vi "Parse Tags - Inline Version.vi"(6 "New Tag Info (F)":bool, 8 "error in (no error)":errorcluster, 9 "[Tags]":string[](array[string]), 11 "Cluster of Controls":variant) -> (0 "error out":errorcluster, 1 "[Whole Tags]":string[](array[string]), 2 "[VData out]":variant[](array[variant]), 3 "[Parsed Tags]":T1[](array[typedef]))   [LabVIEW 2018]
doc: "Converts a variant cluster input and/or an array of references and/or an array of strings to an array of tag information as well as variant data.\nNote1: Empty variant data will be output for Array of Strings.\nNote2: The names/strings will be parsed for any text before the first space in order to find the tags\n\nIf an array of references is input, the VI uses these references to get tag names using the references controls' labels. \n\nIf a cluster of controls is input, each item in the cluster will be used for its label and value.\n\nIf just an array of strings is input, the string values will be used as tags and there will be void values output."
uses:
  Shared Controls/Parsed Tag Cluster.ctl
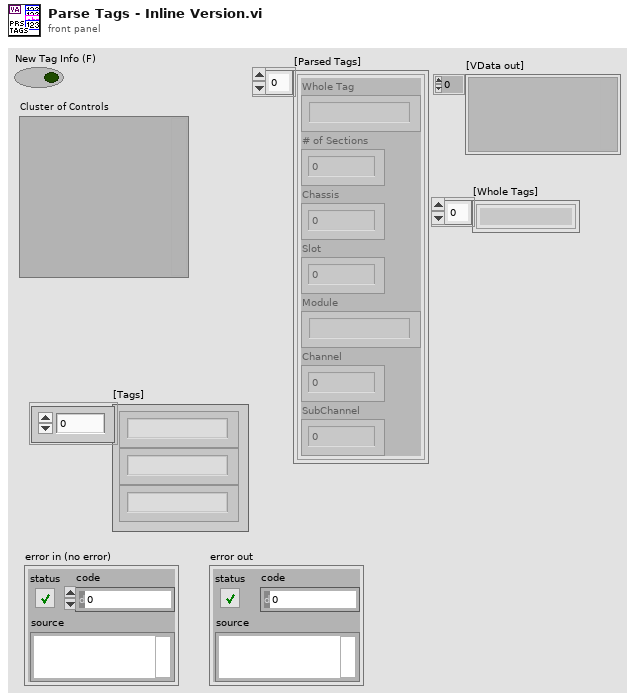
[diagram p1: front panel]
types:
  T1 = typedef "Parsed Tag Cluster.ctl" = cluster{"Whole Tag":string, "# of Sections":u8, "Chassis":u8, "Slot":u8, "Module":string, "Channel":u8, "SubChannel":u8}
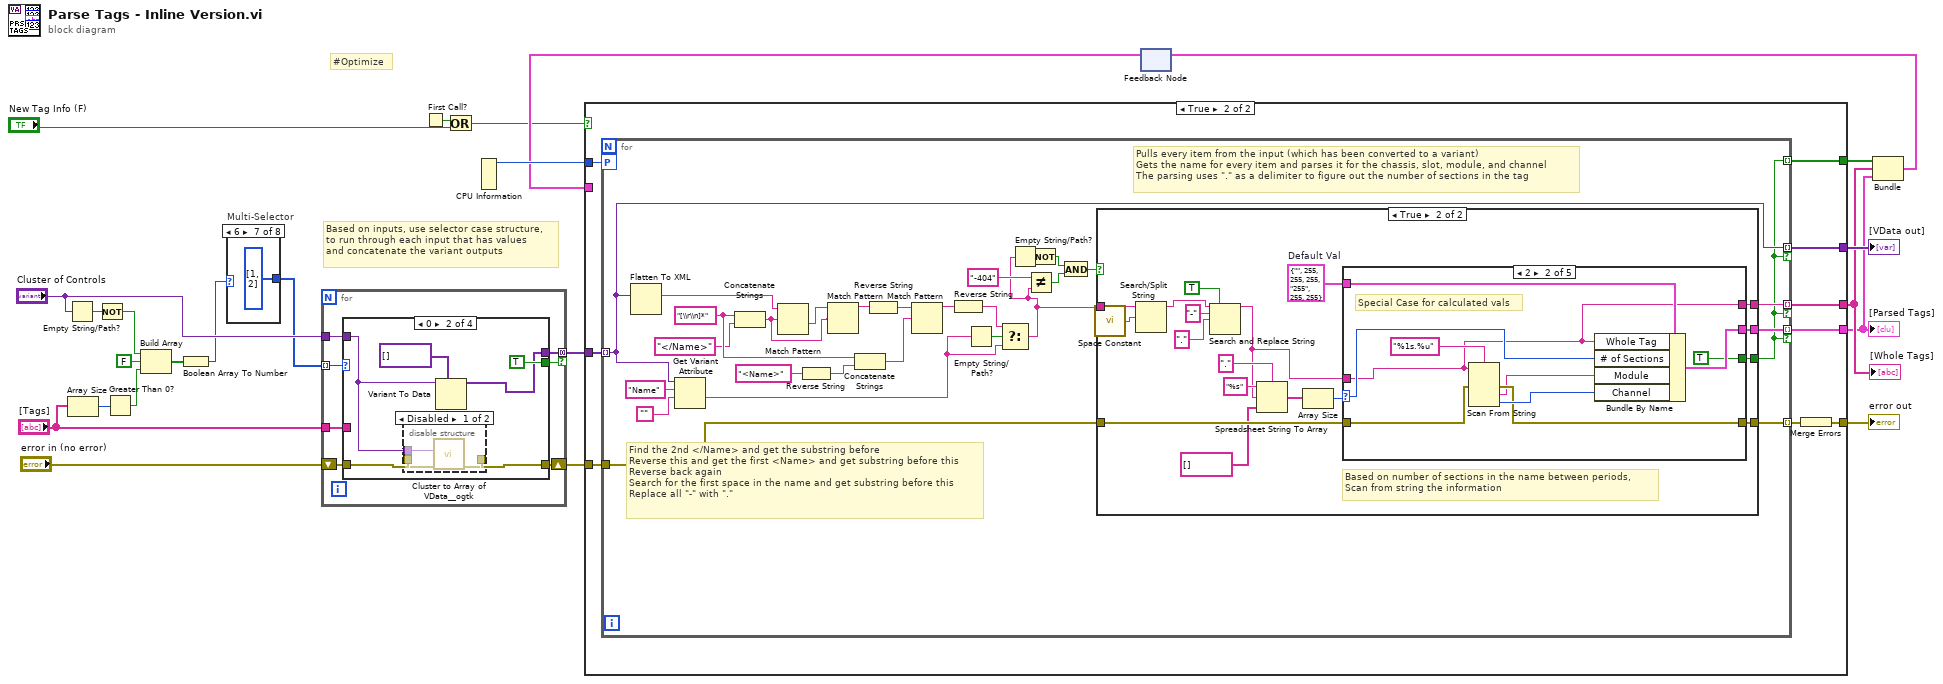
[diagram p0: block diagram]
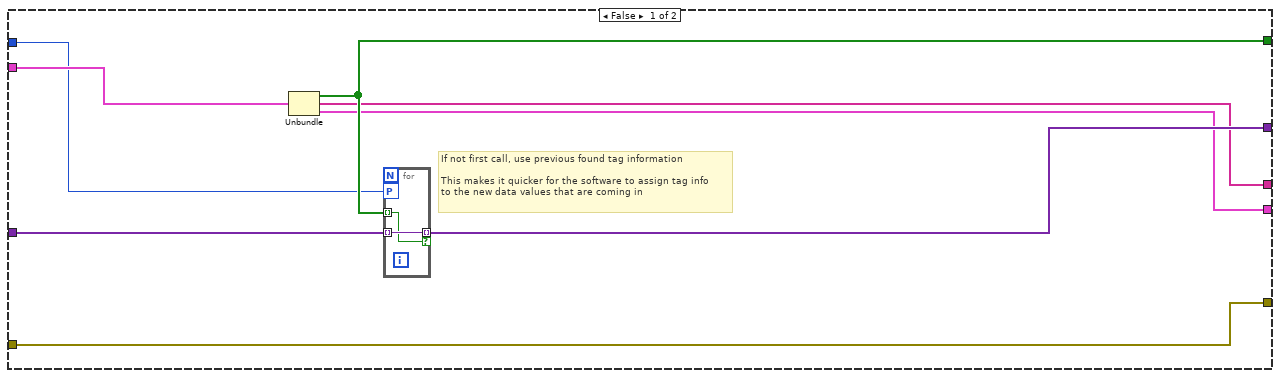
[diagram p2: hidden frame]
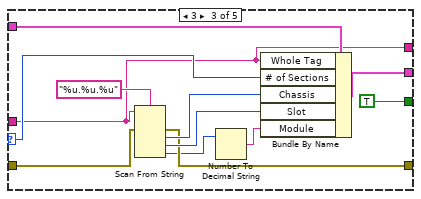
[diagram p5: hidden frame]
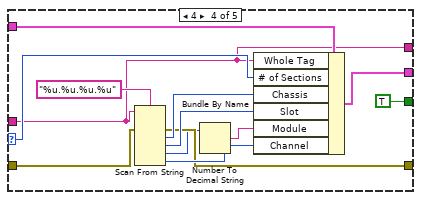
[diagram p6: hidden frame]
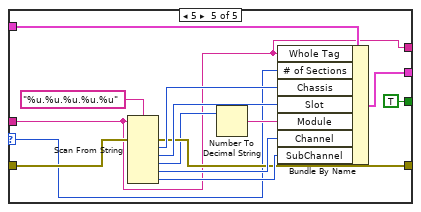
[diagram p7: hidden frame]
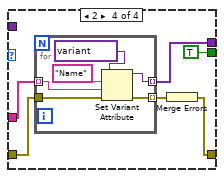
[diagram p11: hidden frame]
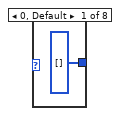
[diagram p12: hidden frame]
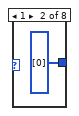
[diagram p13: hidden frame]
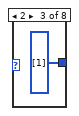
[diagram p14: hidden frame]
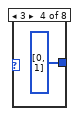
[diagram p15: hidden frame]
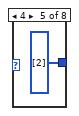
[diagram p16: hidden frame]
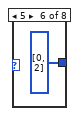
[diagram p17: hidden frame]
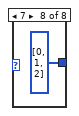
[diagram p18: hidden frame]
diagram:
  # "#Optimize"
  # "Based on inputs, use selector case structure,\nto run through each input that has values\nand concatenate the variant outputs"
  n1 = Empty String/Path?(string/path="Cluster of Controls") -> (empty?=w18:bool)
  n2 = Array Size(array="[Tags]") -> (size(s)=w22:i32)
  n3 = Not(x=w18) -> (.not. x?=w17:bool)
  n4 = Greater Than 0?(x=w22) -> (x > 0?=w21:bool)
  n5 = Build Array(w17, FALSE ("element"), w21) -> (w14:bool[])
  n6 = Boolean Array To Number(Boolean array=w14) -> (number=w16:u32)
  n7 = case "Multi-Selector" shown="6" w16 {
    tunnel: [u32[] [] u32[] [0] u32[] [1] u32[] [0, 1] u32[] [2] u32[] [0, 2] u32[] [1, 2] u32[] [0, 1, 2]] -> w15
    frame 0, Default {
    }
    frame 1 {
    }
    frame 2 {
    }
    frame 3 {
    }
    frame 4 {
    }
    frame 5 {
    }
    frame 6 {
    }
    frame 7 {
    }
  }
  n8 = for {
    tunnel: [w39] -> w24 mode=concatenating if=w33
    tunnel: "[Tags]" -> [w36]
    tunnel: "Cluster of Controls" -> [w35]
    tunnel: w15 -> [w34] mode=indexing
    shift-right: [w37] -> w1
    shift-left: "error in (no error)" -> [w38]
    n9 = case shown="0" w34 {
      tunnel: [_ w41 _ w56] -> w39
      tunnel: w38 -> [w40 w46 w50 w55]
      tunnel: [w40 w45 w50 w52] -> w37
      tunnel: w35 -> [_ w43 _ _]
      tunnel: w36 -> [_ _ _ w53]
      tunnel: [_ TRUE _ TRUE] -> w33
      frame Default {
      }
      frame 0 {
        n10 = disable-structure shown="Disabled" {
          disable-tunnel: w46 -> [w49 _]
          disable-tunnel: [w48 _] -> w45
          disable-tunnel: w43 -> [w47 _]
          frame Disabled {
            n11 = call <userlib>:"Cluster to Array of VData__ogtk.vi"("error in (no error)"=w49, "Cluster"=w47) -> ("error out"=w48:errorcluster)  [unwired: 8 in, 1 out]
          }
          frame Enabled {
          }
        }
        n12 = Variant To Data(type=variant[] [], Variant=w43) -> (data=w41:variant[])  [unwired: 1 in, 1 out]
      }
      frame 1 {
      }
      frame 2 {
        n13 = for {
          tunnel: [w59] -> w56 mode=indexing
          tunnel: w55 -> [w62]
          tunnel: [w61] -> w54 mode=indexing
          tunnel: w53 -> [w58] mode=indexing
          n14 = Set Variant Attribute(Variant=variant(string "TagOnly") ("variant"), name="Name", value=w58, error in=w62) -> (Variant out=w59:variant, error out=w61:errorcluster)  [unwired: 1 out]
        }
        n15 = Merge Errors(w54) -> (w52:errorcluster)
      }
    }
  }
  n16 = First Call?() -> (First Call?: T/F=w11:bool)
  n17 = Or(x=w11, y="New Tag Info (F)") -> (x .or. y?=w5:bool)
  n18 = CPU Information() -> (4:w13:i32)  [unwired: 3 out]
  n19 = feedback #1() -> (w9:cluster{bool[], string[], T1[]})  [unwired: 1 in]
  n20 = case shown="True" w5 {
    tunnel: [w65 w81] -> w6
    tunnel: [w63 w73] -> w3
    tunnel: w24 -> [w70 w80]
    tunnel: w1 -> [w63 w79]
    tunnel: [w69 w78] -> w23
    tunnel: [w66 w77] -> w7
    tunnel: w13 -> [w64 w76]
    tunnel: w9 -> [w68 _]
    tunnel: [w67 w75] -> w10
    frame False {
      # "If not first call, use previous found tag information\n\nThis makes it quicker for the software to assign tag info\nto the new data values that are coming in"
      n21 = Unbundle(w68) -> (w67:bool[], w66:string[], w65:T1[])
      n22 = for {
        tunnel: w70 -> [w72] mode=indexing
        tunnel: [w72] -> w69 mode=indexing if=w71
        tunnel: w67 -> [w71] mode=indexing
        workers-P: w64 -> [_]
      }
    }
    frame True {
      n23 = for {
        tunnel: [w107] -> w81 mode=indexing if=w82
        tunnel: w80 -> [w95] mode=indexing
        tunnel: w79 -> [w109]
        tunnel: [w108] -> w74 mode=indexing
        tunnel: [w95] -> w78 mode=indexing if=w82
        tunnel: [w89] -> w77 mode=indexing if=w82
        workers-P: w76 -> [_]
        tunnel: [w82] -> w75 mode=indexing
        w105 = "[\\r\\n]*"
        # "Find the 2nd </Name> and get the substring before\nReverse this and get the first <Name> and get substring before this\nReverse back again\nSearch for the first space in the name and get substring before this\nReplace all \"-\" with \".\""
        # "Pulls every item from the input (which has been converted to a variant)\nGets the name for every item and parses it for the chassis, slot, module, and channel\nThe parsing uses \".\" as a delimiter to figure out the number of sections in the tag"
        n24 = Flatten To XML(anything=w95) -> (xml string=w102:string)
        n25 = Get Variant Attribute(Variant=w95, name="Name", default value (empty Variant)="") -> (value=w90:string)  [unwired: 1 in, 3 out]
        n26 = Concatenate Strings(w105, "</Name>" ("Substring")) -> (w98:string)
        n27 = Match Pattern(string=w102, regular expression=w98) -> (after substring=w99:string)  [unwired: 1 in, 3 out]
        n28 = Reverse String(1:"<Name>") -> (0:w104:string)
        n29 = Match Pattern(string=w99, regular expression=w98) -> (before substring=w97:string)  [unwired: 1 in, 3 out]
        n30 = Concatenate Strings(w105, w104) -> (w106:string)
        n31 = Reverse String(1:w97) -> (0:w103:string)
        n32 = Match Pattern(string=w103, regular expression=w106) -> (before substring=w96:string)  [unwired: 1 in, 3 out]
        n33 = Reverse String(1:w96) -> (0:w91:string)
        n34 = Empty String/Path?(string/path=w90) -> (empty?=w92:bool)
        n35 = Select(t=w91, s=w92, f=w90) -> (s? t:f=w84:string)
        n36 = Empty String/Path?(string/path=w84) -> (empty?=w86:bool)
        n37 = Not Equal?(x="-404", y=w84) -> (x != y?=w87:bool)
        n38 = Not(x=w86) -> (.not. x?=w88:bool)
        n39 = And(x=w88, y=w87) -> (x .and. y?=w83:bool)
        n40 = case shown="True" w83 {
          tunnel: w109 -> [w110 w127]
          tunnel: [w110 w126] -> w108
          tunnel: [_ w125] -> w107
          tunnel: [_ w113] -> w89
          tunnel: [_ w112] -> w82
          tunnel: w84 -> [_ w111]
          frame False {
          }
          frame True {
            w128 = T1 {"Whole Tag"="", "# of Sections"=255, "Chassis"=255, "Slot"=255, "Module"="255", "Channel"=255, "SubChannel"=255}  # Default Val
            # "Based on number of sections in the name between periods,\nScan from string the information"
            n41 = call <vilib>:"Space Constant.vi"() -> ("String"=w114:string)
            n42 = Search/Split String(string=w111, search string/char (-)=w114) -> (substring before match=w115:string)  [unwired: 1 in, 2 out]
            n43 = Search and Replace String(replace all?=TRUE ("replace all? (F)"), input string=w115, search string="-", replace string="." ("replace string (\"\")")) -> (result string=w119:string)  [unwired: 4 in, 3 out]
            n44 = Spreadsheet String To Array(delimiter (Tab)=".", format string="%s", spreadsheet string=w119, array type (2D Dbl)=string[] []) -> (array=w123:string[])
            n45 = Array Size(array=w123) -> (size(s)=w122:i32)
            n46 = case shown="2" w122 {
              selector: w122 -> [_ w131 w141 w153 w166]
              tunnel: w128 -> [_ w137 w148 w160 w178]
              tunnel: w127 -> [w129 w135 w146 w158 w172]
              tunnel: [w129 w136 w147 w159 w171] -> w126
              tunnel: [_ w134 w143 w155 w167] -> w125
              tunnel: w119 -> [_ w130 w140 w152 w165]
              tunnel: [_ TRUE TRUE TRUE TRUE] -> w112
              tunnel: [_ w130 w140 w152 w165] -> w113
              frame Default {
              }
              frame 2 {
                # "Special Case for calculated vals"
                n47 = Scan From String(format string="%1s.%u" ("regular expression"), input string=w130, error in=w135) -> (error out=w136:errorcluster, output 1=w132:string, output 2=w138:u32)  [unwired: 3 in, 2 out]
                n48 = Bundle By Name(cluster=w137, "Whole Tag"=w130, "# of Sections"=w131, "Module"=w132, "Channel"=w138) -> (w134:T1)
              }
              frame 3 {
                n49 = Scan From String(format string="%u.%u.%u" ("regular expression"), input string=w140, error in=w146) -> (error out=w147:errorcluster, output 1=w150:u32, output 2=w149:u32, output 3=w145:u32)  [unwired: 4 in, 2 out]
                n50 = Number To Decimal String(number=w145) -> (decimal integer string=w144:string)  [unwired: 1 in]
                n51 = Bundle By Name(cluster=w148, "Whole Tag"=w140, "# of Sections"=w141, "Chassis"=w150, "Slot"=w149, "Module"=w144) -> (w143:T1)
              }
              frame 4 {
                n52 = Scan From String(format string="%u.%u.%u.%u" ("regular expression"), input string=w152, error in=w158) -> (error out=w159:errorcluster, output 1=w163:u32, output 2=w162:u32, output 3=w157:u32, output 4=w161:u32)  [unwired: 5 in, 2 out]
                n53 = Number To Decimal String(number=w157) -> (decimal integer string=w156:string)  [unwired: 1 in]
                n54 = Bundle By Name(cluster=w160, "Whole Tag"=w152, "# of Sections"=w153, "Chassis"=w163, "Slot"=w162, "Module"=w156, "Channel"=w161) -> (w155:T1)
              }
              frame 5 {
                n55 = Scan From String(format string="%u.%u.%u.%u.%u" ("regular expression"), input string=w165, error in=w172) -> (error out=w171:errorcluster, output 1=w176:u32, output 2=w175:u32, output 3=w170:u32, output 4=w174:u32, output 5=w173:u32)  [unwired: 6 in, 2 out]
                n56 = Number To Decimal String(number=w170) -> (decimal integer string=w169:string)  [unwired: 1 in]
                n57 = Bundle By Name(cluster=w178, "Whole Tag"=w165, "# of Sections"=w166, "Chassis"=w176, "Slot"=w175, "Module"=w169, "Channel"=w174, "SubChannel"=w173) -> (w167:T1)
              }
            }
          }
        }
      }
      n58 = Merge Errors(w74) -> (w73:errorcluster)
    }
  }
  "[Parsed Tags]" <- w6
  "error out" <- w3
  "[VData out]" <- w23
  "[Whole Tags]" <- w7
  n59 = Bundle(w10, w7, w6) -> (w8:cluster{bool[], string[], T1[]})  [unwired: 1 in]
  n60 = feedback-in #1(w8) -> ()
